vi "AuthSrpInitiationRequest_Create.vi"(7 "Header":T2, 8 "error in (no error)":errorcluster, 9 "AuthSrpInitiationRequest":T1, 11 "ReplyTo":string) -> (0 "error out":errorcluster, 3 "Message":T4)   [LabVIEW 2017]
uses:
  <vilib>/addons/InsightCM/MessageBus/Base/controls/Message.ctl
  <vilib>/addons/InsightCM/MessageBus/Base/controls/MessageHeader.ctl
  <vilib>/addons/InsightCM/MessageBus/Base/controls/KeyValuePair.ctl
  <vilib>/addons/InsightCM/MessageBus/MessageLibrary/Authentication/controls/AuthSrpInitiationRequestBody.ctl
  <vilib>/addons/InsightCM/MessageBus/Base/controls/MessageClassType.ctl
  <vilib>/addons/InsightCM/Utilities/PropertyHelpers/PropertyHelpers.lvlib
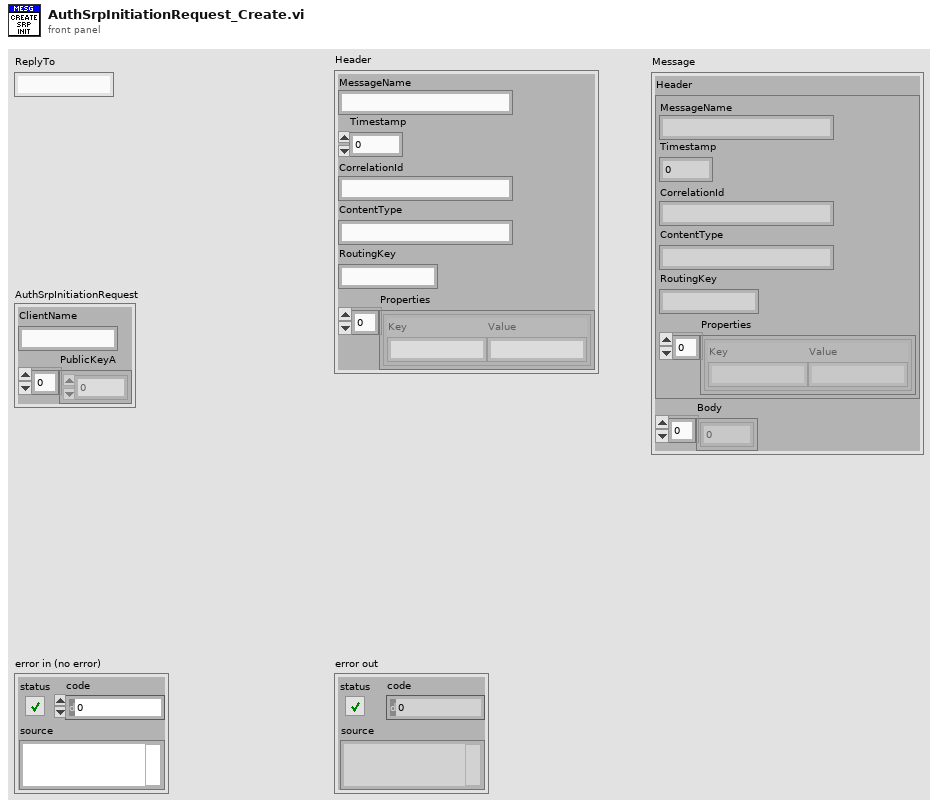
[diagram p1: front panel]
types:
  T1 = typedef "AuthSrpInitiationRequestBody.ctl" = cluster{"ClientName":string, "PublicKeyA":u8[]}
  T2 = typedef "MessageHeader.ctl" = cluster{"MessageName":string, "Timestamp":i64, "CorrelationId":string, "ContentType":string, "RoutingKey":string, "Properties":T3[]}
  T3 = typedef "KeyValuePair.ctl" = cluster{"Key":string, "Value":string}
  T4 = typedef "Message.ctl" = cluster{"Header":T2, "Body":u8[]}
  T5 = cluster{"ClientName":string, "PublicKeyA":string}
  T6 = typedef "MessageClassType.ctl" = enum16{"Request", "Response", "Broadcast", "RoutedMessage"}
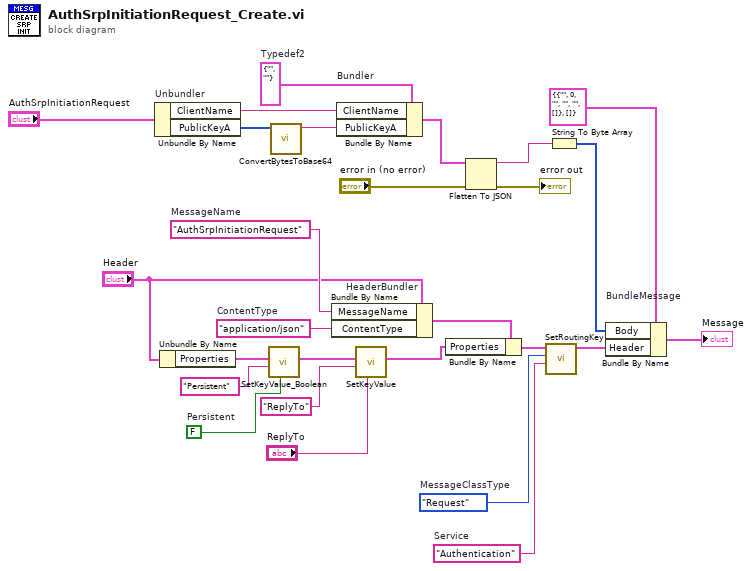
[diagram p0: block diagram]
diagram:
  w4 = T5 {"ClientName"="", "PublicKeyA"=""}  # Typedef2
  w23 = MessageClassType."Request"  # MessageClassType
  w8 = "Authentication"  # Service
  w18 = FALSE  # Persistent
  w24 = "AuthSrpInitiationRequest"  # MessageName
  w21 = "application/json"  # ContentType
  n1 = Unbundle By Name "Unbundler"("AuthSrpInitiationRequest") -> ("ClientName"=w3:string, "PublicKeyA"=w2:u8[])
  n2 = Unbundle By Name("Header") -> ("Properties"=w20:T3[])
  n3 = call <vilib>:"SetKeyValue_Boolean.vi"("value"=w18, "key"="Persistent" ("Key"), "key value pairs"=w20) -> ("key value pairs out"=w16:T3[])  [unwired: 8 in]
  n4 = call <vilib>:"ConvertBytesToBase64.vi"("U8 array"=w2) -> ("base64 encoded"=w1:string)  [unwired: 10 in]
  n5 = Bundle By Name "HeaderBundler"(cluster="Header", "MessageName"=w24, "ContentType"=w21) -> (w14:T2)
  n6 = Bundle By Name "Bundler"(cluster=w4, "ClientName"=w3, "PublicKeyA"=w1) -> (w5:T5)
  n7 = call <vilib>:"SetKeyValue.vi"("value"="ReplyTo", "key"="ReplyTo" ("Key"), "key value pairs"=w16) -> ("key value pairs out"=w13:T3[])  [unwired: 8 in]
  n8 = Bundle By Name(cluster=w14, "Properties"=w13) -> (w15:T2)
  n9 = Flatten To JSON(anything=w5, error in (no error)="error in (no error)") -> (JSON string=w7:string, 11:→"error out":errorcluster)  [unwired: 1 in]
  n10 = call <vilib>:"SetRoutingKey.vi"("SendTo"=w8, "MessageClassType"=w23, "Message Header in"=w15) -> ("Message Header out"=w17:T2)  [unwired: 8 in]
  n11 = String To Byte Array(string=w7) -> (unsigned byte array=w26:u8[])
  n12 = Bundle By Name "BundleMessage"(cluster=T4 {"Header"={"MessageName"="", "Timestamp"=0, "CorrelationId"="", "ContentType"="", "RoutingKey"="", "Properties"=[]}, "Body"=[]} ("Message"), "Body"=w26, "Header"=w17) -> (→"Message":T4)
